vi "Write plot data.vi"(8 "error in (no error)":errorcluster, 10 "plot data":cluster{"X":dbl, "Y":dbl, "flag":u8}[](array[cluster]), 11 "Plots in":refnum<class "Plots.lvclass">) -> (0 "error out":errorcluster, 3 "Plots out":refnum<class "Plots.lvclass">)   [LabVIEW 2018, in "Plots.lvclass"]
uses:
  Plots.lvclass
  Plots.lvclass/Plots.ctl
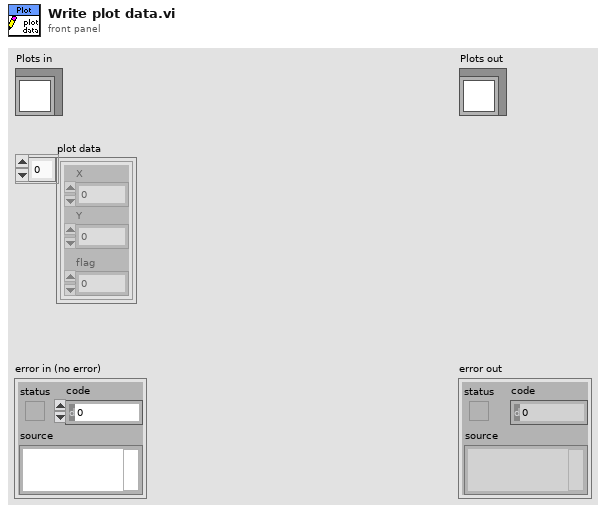
[diagram p1: front panel]
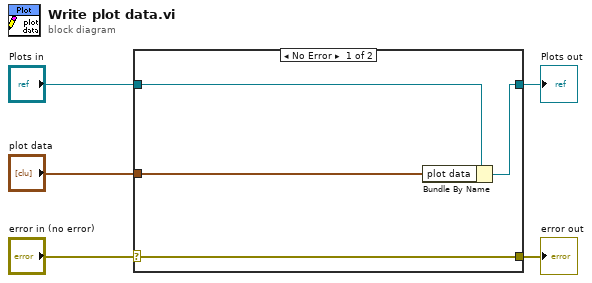
[diagram p0: block diagram]
diagram:
  n1 = case shown="No Error" "error in (no error)" {
    selector: "error in (no error)" -> [w9 w10]
    tunnel: [w9 w10] -> w4
    tunnel: [w7 w11] -> w2
    tunnel: "Plots in" -> [w8 w11]
    tunnel: "plot data" -> [w6 _]
    frame No Error {
      n2 = Bundle By Name(cluster=w8, "plot data"=w6) -> (w7:refnum<class "Plots.lvclass">)
    }
    frame Error {
    }
  }
  "error out" <- w4
  "Plots out" <- w2
